vi "Get Measurement (Multiple).vi"(8 "error in (no error)":errorcluster, 9 "Measurement Names":string, 10 "IED Names":string, 11 "SCADA in":refnum<class "SCADA.lvclass">) -> (0 "error out":errorcluster, 3 "SCADA out":refnum<class "SCADA.lvclass">)   [LabVIEW 2015, in "SCADA Core.lvlib" / "SCADA.lvclass"]
doc: "This takes a comma-delimited list of IED Names and Measurement Names and returns the measurements as a double array flattened to a string."
uses:
  SCADA.lvclass
  <vilib>/ActorFramework/Actor/Actor.lvclass/Actor.ctl
  SCADA.lvclass/SCADA.ctl
  SCADA Abstract Messages/IED Measurement Status Msg/IED Measurement Status.ctl
  <vilib>/NI/Tools/Keyed Array/Map String.vi
  <vilib>/NI/Tools/String/Get Case Matching.vi
  <vilib>/NI/Tools/Keyed Array/Tools_KeyedArray.lvlib
  <vilib>/ActorFramework/Actor/Actor.lvclass
  SCADA Abstract Messages/IED Measurement Status Msg/IED Measurement Status Msg.lvclass
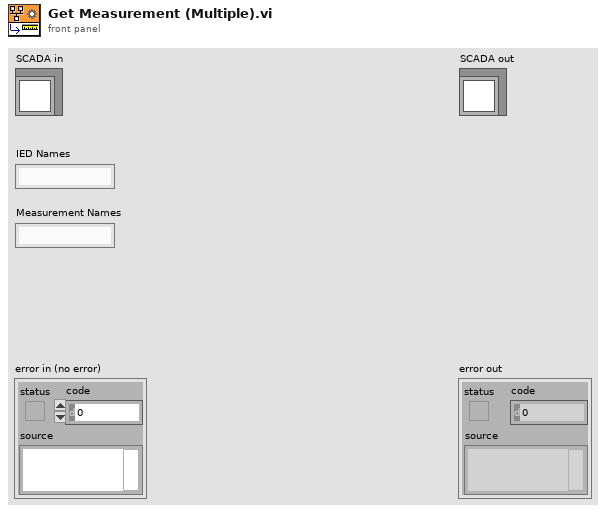
[diagram p1: front panel]
types:
  T1 = typedef "SCADA Core.lvlib/IED Measurement Status Msg.lvclass/IED Measurement Status.ctl" = enum16{"Single Success", "Single Failure", "Multiple Success", "Multiple Failure"}
  T2 = typedef "Tools_KeyedArray.lvlib/KeyedArray.ctl" = cluster{"keys":string[], "values":string[]}
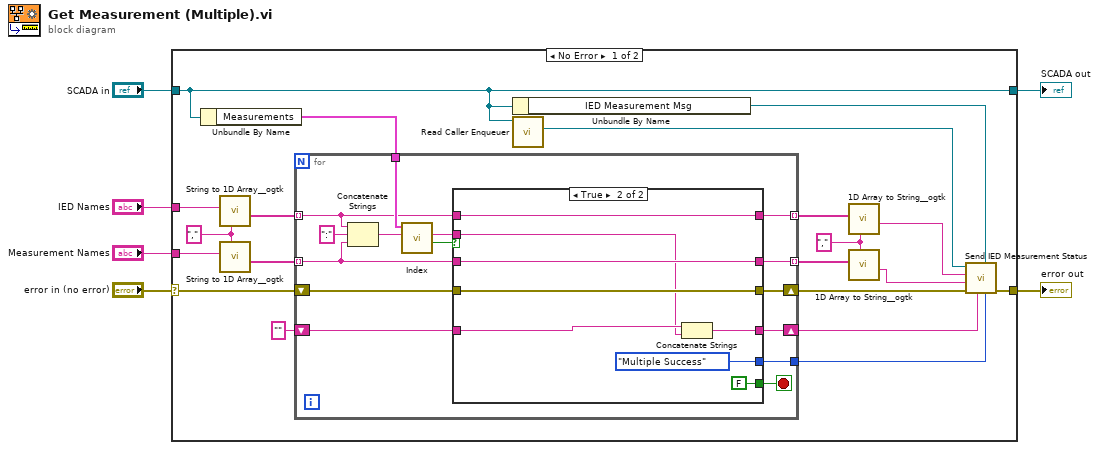
[diagram p0: block diagram]
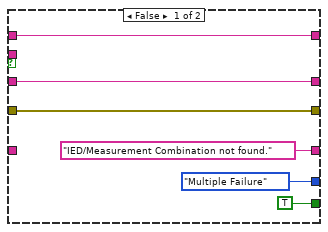
[diagram p2: hidden frame]
diagram:
  n1 = case shown="No Error" "error in (no error)" {
    selector: "error in (no error)" -> [w25 w57]
    tunnel: [w20 w57] -> w5
    tunnel: [w24 w56] -> w3
    tunnel: "SCADA in" -> [w24 w56]
    tunnel: "IED Names" -> [w18 _]
    tunnel: "Measurement Names" -> [w16 _]
    frame No Error {
      w10 = "," ("delimiter (Tab)")
      w14 = "," ("delimiter (Tab)")
      n2 = Unbundle By Name(w24) -> ("Measurements"=w26:T2)
      n3 = call <userlib>:"String to 1D Array__ogtk.vi"("delimiter (Tab)"=w14, "string"=w18) -> ("Array of Strings"=w17:string[])  [unwired: 9 in]
      n4 = call <userlib>:"String to 1D Array__ogtk.vi"("delimiter (Tab)"=w14, "string"=w16) -> ("Array of Strings"=w15:string[])  [unwired: 9 in]
      n5 = for {
        tunnel: w26 -> [w40]
        tunnel: [w34] -> w19
        tunnel: [w32] -> w13 mode=indexing
        tunnel: [w31] -> w11 mode=indexing
        tunnel: w17 -> [w30] mode=indexing
        tunnel: w15 -> [w29] mode=indexing
        shift-right: [w35] -> w21
        shift-left: w25 -> [w37]
        shift-right: [w33] -> w7
        shift-left: "" ("value") -> [w27]
        stop <- w28 stop-if-true
        n6 = Concatenate Strings(w30, ":" ("string"), w29) -> (w39:string)
        n7 = call <vilib>:"Index.vi"("key"=w39, "array in"=w40) -> ("valid key"=w38:bool, "value"=w36:string)  [unwired: 3 in, 1 out]
        n8 = case shown="True" w38 {
          tunnel: w37 -> [w47 w55]
          tunnel: w36 -> [_ w49]
          tunnel: w30 -> [w46 w53]
          tunnel: w29 -> [w45 w52]
          tunnel: [w47 w55] -> w35
          tunnel: [IED_Measurement_Status."Multiple Failure" ("Status") IED_Measurement_Status."Multiple Success" ("Status")] -> w34
          tunnel: ["IED/Measurement Combination not found." ("value") w48] -> w33
          tunnel: [w46 w53] -> w32
          tunnel: [w45 w52] -> w31
          tunnel: [TRUE FALSE] -> w28
          tunnel: w27 -> [_ w50]
          frame False {
          }
          frame True {
            n9 = Concatenate Strings(w50, w49) -> (w48:string)
          }
        }
      }
      n10 = Unbundle By Name(w24) -> ("IED Measurement Msg"=w23:refnum<class "IED Measurement Status Msg.lvclass">)
      n11 = call <vilib>:"Read Caller Enqueuer.vi"("Actor"=w24) -> ("Caller Enqueuer"=w22:refnum<class "Message Enqueuer.lvclass">)  [unwired: 10 in]
      n12 = call <userlib>:"1D Array to String__ogtk.vi"("delimiter (Tab)"=w10, "Array of Strings"=w13) -> ("delimited string"=w12:string)  [unwired: 9 in]
      n13 = call <userlib>:"1D Array to String__ogtk.vi"("delimiter (Tab)"=w10, "Array of Strings"=w11) -> ("delimited string"=w9:string)  [unwired: 9 in]
      n14 = call "Send IED Measurement Status.vi"("Status"=w19, "IED Measurement Msg"=w23, "Value/error"=w7, "error in (no error)"=w21, "Measurement Name"=w9, "IED Name"=w12, "Message Enqueuer in"=w22) -> ("error out"=w20:errorcluster)  [unwired: 3 in, 1 out]
    }
    frame Error {
    }
  }
  "error out" <- w5
  "SCADA out" <- w3
